vi "my_read_data.vi"   [LabVIEW 2020]
types:
  T1 = enum16{"big-endian, network order", "native, host order", "little-endian"}
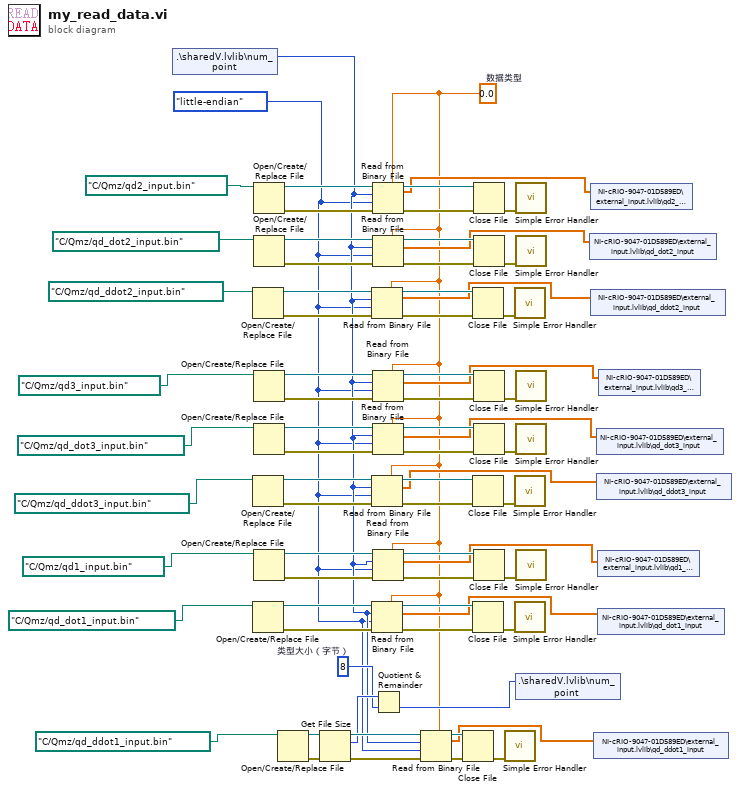
[diagram p0: block diagram]
diagram:
  w7 = i64 8  # 类型大小（字节）
  w5 = 0.0  # 数据类型
  w2 = T1."little-endian" ("字节顺序(0:big-endian, network order)")
  n1 = shared-variable ".\\sharedV.lvlib\\num_point"() -> (w3:i32)  [unwired: 1 in, 1 out]
  n2 = Open/Create/Replace File(file path (use dialog)=path "C:/Qmz/qd_ddot2_input.bin") -> (refnum out=w56:refnum<file>, error out=w57:errorcluster)  [unwired: 5 in, 1 out]
  n3 = Open/Create/Replace File(file path (use dialog)=path "C:/Qmz/qd_ddot3_input.bin") -> (refnum out=w37:refnum<file>, error out=w38:errorcluster)  [unwired: 5 in, 1 out]
  n4 = Open/Create/Replace File(file path (use dialog)=path "C:/Qmz/qd_dot1_input.bin") -> (refnum out=w23:refnum<file>, error out=w24:errorcluster)  [unwired: 5 in, 1 out]
  n5 = Open/Create/Replace File(file path (use dialog)=path "C:/Qmz/qd2_input.bin") -> (refnum out=w67:refnum<file>, error out=w69:errorcluster)  [unwired: 5 in, 1 out]
  n6 = Open/Create/Replace File(file path (use dialog)=path "C:/Qmz/qd_dot2_input.bin") -> (refnum out=w61:refnum<file>, error out=w63:errorcluster)  [unwired: 5 in, 1 out]
  n7 = Open/Create/Replace File(file path (use dialog)=path "C:/Qmz/qd3_input.bin") -> (refnum out=w47:refnum<file>, error out=w48:errorcluster)  [unwired: 5 in, 1 out]
  n8 = Open/Create/Replace File(file path (use dialog)=path "C:/Qmz/qd_dot3_input.bin") -> (refnum out=w42:refnum<file>, error out=w43:errorcluster)  [unwired: 5 in, 1 out]
  n9 = Open/Create/Replace File(file path (use dialog)=path "C:/Qmz/qd1_input.bin") -> (refnum out=w20:refnum<file>, error out=w27:errorcluster)  [unwired: 5 in, 1 out]
  n10 = Open/Create/Replace File(file path (use dialog)=path "C:/Qmz/qd_ddot1_input.bin") -> (refnum out=w10:refnum<file>, error out=w13:errorcluster)  [unwired: 5 in, 1 out]
  n11 = Get File Size(file=w10, error in=w13) -> (refnum out=w9:refnum<file>, size (in bytes)=w8:i64, 0:w14:errorcluster)
  n12 = Read from Binary File(5:w5, 8:w57, 9:w2, 10:w3, 11:w56) -> (0:w59:errorcluster, 2:w51:dbl[], 3:w55:refnum<file>)  [unwired: 1 in, 1 out]
  n13 = Read from Binary File(5:w5, 8:w38, 9:w2, 10:w3, 11:w37) -> (0:w40:errorcluster, 2:w30:dbl[], 3:w36:refnum<file>)  [unwired: 1 in, 1 out]
  n14 = Read from Binary File(5:w5, 8:w24, 9:w2, 10:w3, 11:w23) -> (0:w26:errorcluster, 2:w16:dbl[], 3:w22:refnum<file>)  [unwired: 1 in, 1 out]
  n15 = Read from Binary File(5:w5, 8:w69, 9:w2, 10:w3, 11:w67) -> (0:w71:errorcluster, 2:w53:dbl[], 3:w66:refnum<file>)  [unwired: 1 in, 1 out]
  n16 = Read from Binary File(5:w5, 8:w63, 9:w2, 10:w3, 11:w61) -> (0:w65:errorcluster, 2:w52:dbl[], 3:w60:refnum<file>)  [unwired: 1 in, 1 out]
  n17 = Read from Binary File(5:w5, 8:w48, 9:w2, 10:w3, 11:w47) -> (0:w50:errorcluster, 2:w32:dbl[], 3:w46:refnum<file>)  [unwired: 1 in, 1 out]
  n18 = Read from Binary File(5:w5, 8:w43, 9:w2, 10:w3, 11:w42) -> (0:w45:errorcluster, 2:w31:dbl[], 3:w41:refnum<file>)  [unwired: 1 in, 1 out]
  n19 = Read from Binary File(5:w5, 8:w27, 9:w2, 10:w3, 11:w20) -> (0:w29:errorcluster, 2:w17:dbl[], 3:w19:refnum<file>)  [unwired: 1 in, 1 out]
  n20 = Quotient & Remainder(x=w8, y=w7) -> (floor(x/y)=w6:i64)  [unwired: 1 out]
  n21 = Read from Binary File(5:w5, 8:w14, 9:w2, 10:w3, 11:w9) -> (0:w15:errorcluster, 2:w1:dbl[], 3:w4:refnum<file>)  [unwired: 1 in, 1 out]
  n22 = Close File(refnum=w4, error in=w15) -> (error out=w12:errorcluster)  [unwired: 1 out]
  n23 = Close File(refnum=w55, error in=w59) -> (error out=w58:errorcluster)  [unwired: 1 out]
  n24 = Close File(refnum=w36, error in=w40) -> (error out=w39:errorcluster)  [unwired: 1 out]
  n25 = Close File(refnum=w22, error in=w26) -> (error out=w25:errorcluster)  [unwired: 1 out]
  n26 = Close File(refnum=w66, error in=w71) -> (error out=w70:errorcluster)  [unwired: 1 out]
  n27 = Close File(refnum=w60, error in=w65) -> (error out=w64:errorcluster)  [unwired: 1 out]
  n28 = Close File(refnum=w46, error in=w50) -> (error out=w49:errorcluster)  [unwired: 1 out]
  n29 = Close File(refnum=w41, error in=w45) -> (error out=w44:errorcluster)  [unwired: 1 out]
  n30 = Close File(refnum=w19, error in=w29) -> (error out=w28:errorcluster)  [unwired: 1 out]
  n31 = call <vilib>:"Simple Error Handler.vi"("error in (no error)"=w12) -> ()  [unwired: 4 in, 5 out]
  n32 = call <vilib>:"Simple Error Handler.vi"("error in (no error)"=w58) -> ()  [unwired: 4 in, 5 out]
  n33 = call <vilib>:"Simple Error Handler.vi"("error in (no error)"=w39) -> ()  [unwired: 4 in, 5 out]
  n34 = call <vilib>:"Simple Error Handler.vi"("error in (no error)"=w25) -> ()  [unwired: 4 in, 5 out]
  n35 = call <vilib>:"Simple Error Handler.vi"("error in (no error)"=w70) -> ()  [unwired: 4 in, 5 out]
  n36 = call <vilib>:"Simple Error Handler.vi"("error in (no error)"=w64) -> ()  [unwired: 4 in, 5 out]
  n37 = call <vilib>:"Simple Error Handler.vi"("error in (no error)"=w49) -> ()  [unwired: 4 in, 5 out]
  n38 = call <vilib>:"Simple Error Handler.vi"("error in (no error)"=w44) -> ()  [unwired: 4 in, 5 out]
  n39 = call <vilib>:"Simple Error Handler.vi"("error in (no error)"=w28) -> ()  [unwired: 4 in, 5 out]
  n40 = shared-variable ".\\sharedV.lvlib\\num_point"(w6) -> ()  [unwired: 1 in, 1 out]
  n41 = shared-variable "NI-cRIO-9047-01D589ED\\external_input.lvlib\\qd_dot2_input"(w52) -> ()  [unwired: 1 in, 1 out]
  n42 = shared-variable "NI-cRIO-9047-01D589ED\\external_input.lvlib\\qd2_input"(w53) -> ()  [unwired: 1 in, 1 out]
  n43 = shared-variable "NI-cRIO-9047-01D589ED\\external_input.lvlib\\qd_ddot2_input"(w51) -> ()  [unwired: 1 in, 1 out]
  n44 = shared-variable "NI-cRIO-9047-01D589ED\\external_input.lvlib\\qd_ddot1_input"(w1) -> ()  [unwired: 1 in, 1 out]
  n45 = shared-variable "NI-cRIO-9047-01D589ED\\external_input.lvlib\\qd_dot3_input"(w31) -> ()  [unwired: 1 in, 1 out]
  n46 = shared-variable "NI-cRIO-9047-01D589ED\\external_input.lvlib\\qd_ddot3_input"(w30) -> ()  [unwired: 1 in, 1 out]
  n47 = shared-variable "NI-cRIO-9047-01D589ED\\external_input.lvlib\\qd1_input"(w17) -> ()  [unwired: 1 in, 1 out]
  n48 = shared-variable "NI-cRIO-9047-01D589ED\\external_input.lvlib\\qd_dot1_input"(w16) -> ()  [unwired: 1 in, 1 out]
  n49 = shared-variable "NI-cRIO-9047-01D589ED\\external_input.lvlib\\qd3_input"(w32) -> ()  [unwired: 1 in, 1 out]
